vi "Tank.vi"() -> ()   [LabVIEW 2016]
uses:
  Pathfinder-Lib/VIs/Waypoint.ctl
  Pathfinder-Lib/Pathfinder.lvlib
panel:
  in  "Tab Control":enum32{"Primary Path", "Tank Position"}(tab)=enum."Tank Position"
  out "Path":T1(graph)
  out "Position":cluster{dbl[], dbl[]}[](graph)
  out "error out":errorcluster
  in  "wheelbase_width":dbl=24.0
  in  "sample_count":i32=1000
  in  "dt":dbl=0.001
  in  "max_jerk":dbl=60.0
  in  "max_acceleration":dbl=10.0
  in  "max_velocity":dbl=15.0
  in  "path":T2[](array[typedef])=[{"x"=12.0, "y"=60.0, "angle"=0.0}, {"x"=132.0, "y"=125.0, "angle"=60.0}]
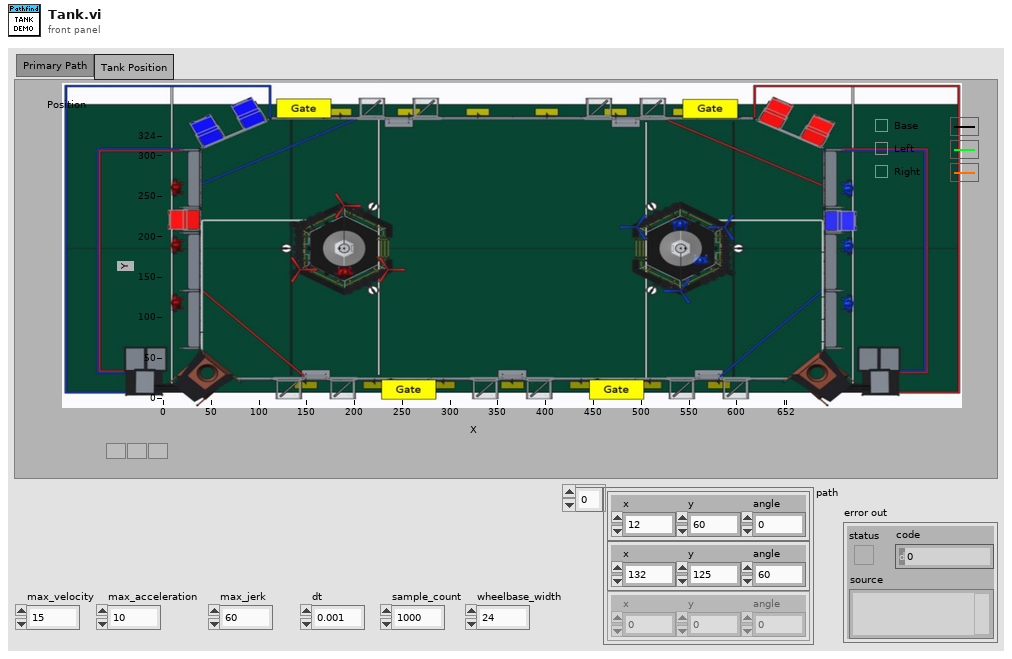
[diagram p1: front panel]
types:
  T1 = cluster{"position":dbl, "velocity":dbl, "acceleration":dbl, "jerk":dbl, "heading":dbl}[]
  T2 = typedef "Pathfinder.lvlib/Waypoint.ctl" = cluster{"x":dbl, "y":dbl, "angle":dbl}
  T3 = typedef "Pathfinder.lvlib/Segment.ctl" = cluster{"dt":dbl, "x":dbl, "y":dbl, "position":dbl, "velocity":dbl, "acceleration":dbl, "jerk":dbl, "heading":dbl}
  T4 = cluster{"position":dbl, "velocity":dbl, "acceleration":dbl, "jerk":dbl, "heading":dbl}
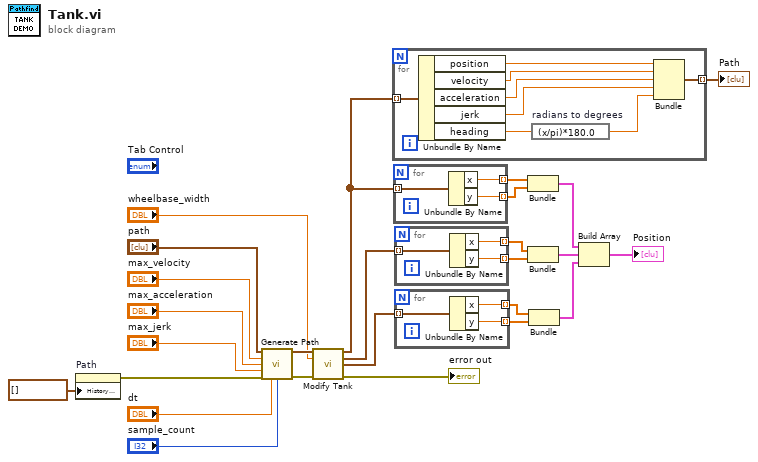
[diagram p0: block diagram]
diagram:
  n1 = property on="Path" class="WFChart (strict)"("History Data"=T1 []) -> (error out=w2:errorcluster)  [unwired: 2 in, 1 out]
  n2 = call "Generate Path.vi"("path"="path", "max_velocity"="max_velocity", "max_acceleration"="max_acceleration", "max_jerk"="max_jerk", "error in"=w2, "dt (.001)"="dt", "sample_count (100000)"="sample_count") -> ("Segments"=w26:T3[], "error out"=w21:errorcluster)  [unwired: 7 in]
  n3 = call "Modify Tank.vi"("Original"=w26, "wheelbase_width"="wheelbase_width", "error in"=w21) -> ("original"=w7:T3[], "left"=w16:T3[], "right"=w15:T3[], "error out"=→"error out":errorcluster)  [unwired: 9 in]
  n4 = for {
    tunnel: w7 -> [w34] mode=indexing
    tunnel: [w28] -> w17 mode=indexing
    n5 = Unbundle By Name(w34) -> ("position"=w33:dbl, "velocity"=w32:dbl, "acceleration"=w31:dbl, "jerk"=w30:dbl, "heading"=w29:dbl)
    n6 = expression code="(x/pi)*180.0" "radians to degrees"(w29) -> (w27:dbl)
    n7 = Bundle("position"=w33, "velocity"=w32, "acceleration"=w31, "jerk"=w30, "heading"=w27) -> (w28:T4)  [unwired: 1 in]
  }
  "Path" <- w17
  n8 = for {
    tunnel: w7 -> [w37] mode=indexing
    tunnel: [w36] -> w6 mode=indexing
    tunnel: [w35] -> w5 mode=indexing
    n9 = Unbundle By Name(w37) -> ("x"=w36:dbl, "y"=w35:dbl)
  }
  n10 = for {
    tunnel: w16 -> [w40] mode=indexing
    tunnel: [w39] -> w14 mode=indexing
    tunnel: [w38] -> w13 mode=indexing
    n11 = Unbundle By Name(w40) -> ("x"=w39:dbl, "y"=w38:dbl)
  }
  n12 = for {
    tunnel: w15 -> [w43] mode=indexing
    tunnel: [w42] -> w12 mode=indexing
    tunnel: [w41] -> w11 mode=indexing
    n13 = Unbundle By Name(w43) -> ("x"=w42:dbl, "y"=w41:dbl)
  }
  n14 = Bundle(w6, w5) -> (w4:cluster{dbl[], dbl[]})  [unwired: 1 in]
  n15 = Bundle(w14, w13) -> (w9:cluster{dbl[], dbl[]})  [unwired: 1 in]
  n16 = Bundle(w12, w11) -> (w10:cluster{dbl[], dbl[]})  [unwired: 1 in]
  n17 = Build Array(w4, w9, w10) -> (→"Position":cluster{dbl[], dbl[]}[])
